vi "Teleop V1.vi"(10 "Match Info":T1={"Autonomous Elapsed Seconds"=0.0, "TeleOp Elapsed Seconds"=567.647, "Disabled Elapsed Seconds"=48.494, "Visited Autonomous"=FALSE, "Visited TeleOp"=TRUE, "Visited Disabled"=TRUE, "Autonomous Settings"={"Autonomous Style"=enum."Independent", "VI Refnum"=refnum}}) -> ()   [LabVIEW 2018]
doc: "This VI is called for each TeleOp packet received from the DS where the robot is not disabled. It is often used to read from the joysticks and update I/O or to update setpoints for timed control loops. It should complete and return within 20 milliseconds or it may miss DS packets."
uses:
  <vilib>/Rock Robotics/WPI/DriverStation/WPI_DriverStationMatch Info.ctl
  <vilib>/Rock Robotics/WPI/Solenoid/WPI_SolenoidValue.ctl
  <vilib>/Rock Robotics/WPI/ThirdParty/Phoenix-LabVIEW/Motor Controller/Controls/CTRE_Phoenix_MotorControl_ControlMode.ctl
  Refnums.vi
  <vilib>/Rock Robotics/Network Tables/NT Write Numeric Array.vi
  <vilib>/Rock Robotics/Network Tables/NT Write Boolean Array.vi
  <vilib>/Rock Robotics/WPI/Solenoid/WPI_SolenoidSetEnum.vi
  <vilib>/Rock Robotics/WPI/ThirdParty/Phoenix-LabVIEW/Motor Controller/Get/CTRE_Phoenix_MotorController_GetQuadratureData.vi
  Various Globals.vi
panel:
  out "Climber Position":dbl=-130.0
  in  "Elevator cargo":dbl=10500.0
  in  "Elevator First Level":dbl=5500.0
  in  "Pivot Under Flat":dbl=1300.0
  in  "Climber Clear 2":dbl=-300.0
  out "Boolean":bool=TRUE
  out "Pivot Position":dbl=64.0
  out "Elevator Position":dbl=439.0
  in  "Random Climber":dbl=2000.0
  in  "Climber Climb":dbl=5500.0
  in  "Elevator Tucked":dbl=500.0
  in  "Pivot Up":dbl
  in  "Elevator Intake":dbl=500.0
  in  "Climber Clear":dbl=1500.0
  in  "Elevator Clearance":dbl=4750.0
  in  "Pivot Intake":dbl=1650.0
  in  "Second level":dbl=14500.0
  in  "First Ball":dbl=7500.0
  in  "Climber Intake":dbl=2700.0
  in  "Climber Up":dbl
  # "Climber Intake \nChanged From\n2800"
  # "<---- Changed From 1700"
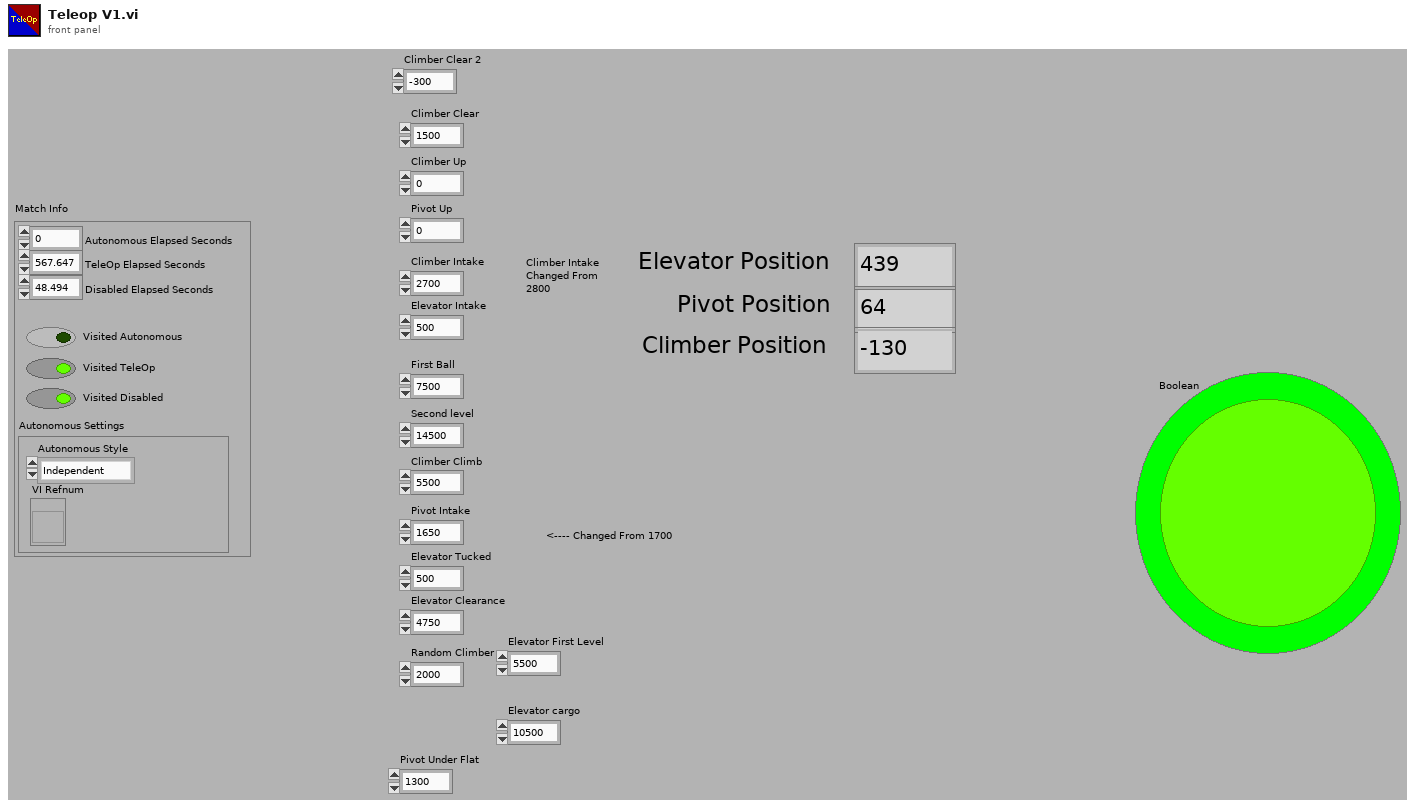
[diagram p1: front panel]
types:
  T1 = typedef "WPI_DriverStationMatch Info.ctl" = cluster{"Autonomous Elapsed Seconds":dbl, "TeleOp Elapsed Seconds":dbl, "Disabled Elapsed Seconds":dbl, "Visited Autonomous":bool, "Visited TeleOp":bool, "Visited Disabled":bool, "Autonomous Settings":cluster{"Autonomous Style":enum16{"Iterative", "Independent"}, "VI Refnum":refnum<vi>}}
  T2 = typedef "WPI_JoystickDevRef.ctl" = cluster{"Device":T3}
  T3 = typedef "WPI_JoystickDeviceEnum.ctl" = enum16{"USB 0", "USB 1", "USB 2", "USB 3", "USB 4", "USB 5"}
  T4 = typedef "WPI_RobotDriveDevRef.ctl" = cluster{"DevStatus":errorcluster, "Motors[]":T5[], "Square Inputs":bool, "Max Output":dbl}
  T5 = typedef "WPI_MotorControlDeviceRef.ctl" = cluster{"DeviceStatus":errorcluster, "Type":T6, "PWM":cluster{"PWM Channel":T7, "DeadBand":T8}, "CAN":cluster{"Device Number":u8, "SetOutput VI Ref":variant, "GetOutput VI Ref":variant, "Enable VI Ref":variant, "Disable VI Ref":variant, "Data":variant}, "Invert":bool, "DIO PWM":cluster{"PWM \"Enable\" Channel":T7, "DIOChannel":T9, "PWM Rate":dbl}}
  T6 = typedef "WPI_MotorControlType.ctl" = enum16{"PWM", "CAN", "DIO PWM"}
  T7 = typedef "FPGA_DIOPWMChannel.ctl" = enum8{"PWM 0", "PWM 1", "PWM 2", "PWM 3", "PWM 4", "PWM 5", "PWM 6", "PWM 7", "PWM 8", "PWM 9", "PWM MXP 0", "PWM MXP 1", "PWM MXP 2", "PWM MXP 3", "PWM MXP 4", "PWM MXP 5", "PWM MXP 6", "PWM MXP 7", "PWM MXP 8", "PWM MXP 9", "Invalid"}
  T8 = typedef "WPI_PWMDeadband.ctl" = cluster{"Name":string, "maxPositivePwm":i32, "minPositivePwm":i32, "centerPwm":i32, "maxNegativePwm":i32, "minNegativePwm":i32, "angularRange":u16}
  T9 = typedef "FPGA_DIOChannel.ctl" = enum8{"DIO 0", "DIO 1", "DIO 2", "DIO 3", "DIO 4", "DIO 5", "DIO 6", "DIO 7", "DIO 8", "DIO 9", "DIO MXP 0", "DIO MXP 1", "DIO MXP 2", "DIO MXP 3", "DIO MXP 4", "DIO MXP 5", "DIO MXP 6", "DIO MXP 7", "DIO MXP 8", "DIO MXP 9", "DIO MXP 10", "DIO MXP 11", "DIO MXP 12", "DIO MXP 13", "DIO MXP 14", "DIO MXP 15", "SPI Port CS1", "SPI Port CS2", "SPI Port CS3", "SPI Port MISO", "SPI Port MOSI", "Invalid"}
  T10 = cluster{"DriveTrain":T4, "LeftDrive":T5, "RightDrive":T5, "Elevator":T5, "Pivot":T5, "Intake":T5, "Right Climber":T5, "Left Climber":T5, "Shooter":T5}
  T11 = typedef "WPI_SolenoidDevRef.ctl" = cluster{"DevStatus":errorcluster, "Pneumatics Control Module":u8, "Forward Solenoid Channel":T12, "Reverse Solenoid Channel":T12}
  T12 = typedef "WPI_SolenoidChannel.ctl" = enum8{"Solenoid 0", "Solenoid 1", "Solenoid 2", "Solenoid 3", "Solenoid 4", "Solenoid 5", "Solenoid 6", "Solenoid 7", "Invalid"}
  T13 = typedef "WPI_CompressorDevRef.ctl" = cluster{"DevStatus":errorcluster, "Pneumatics Control Module":u8}
  T14 = cluster{"DriveShifter":T11, "Ouput":T11, "Compressor":T13, "Climb Piston":T11}
  T15 = typedef "WPI_SolenoidValue.ctl" = enum16{"Off", "On", "Forward", "Reverse"}
  T16 = typedef "WPI_DigitalInputDevRef.ctl" = cluster{"DevStatus":errorcluster, "DIO Channel":T9}
  T17 = typedef "CTRE_Phoenix_MotorControl_ControlMode.ctl" = u16
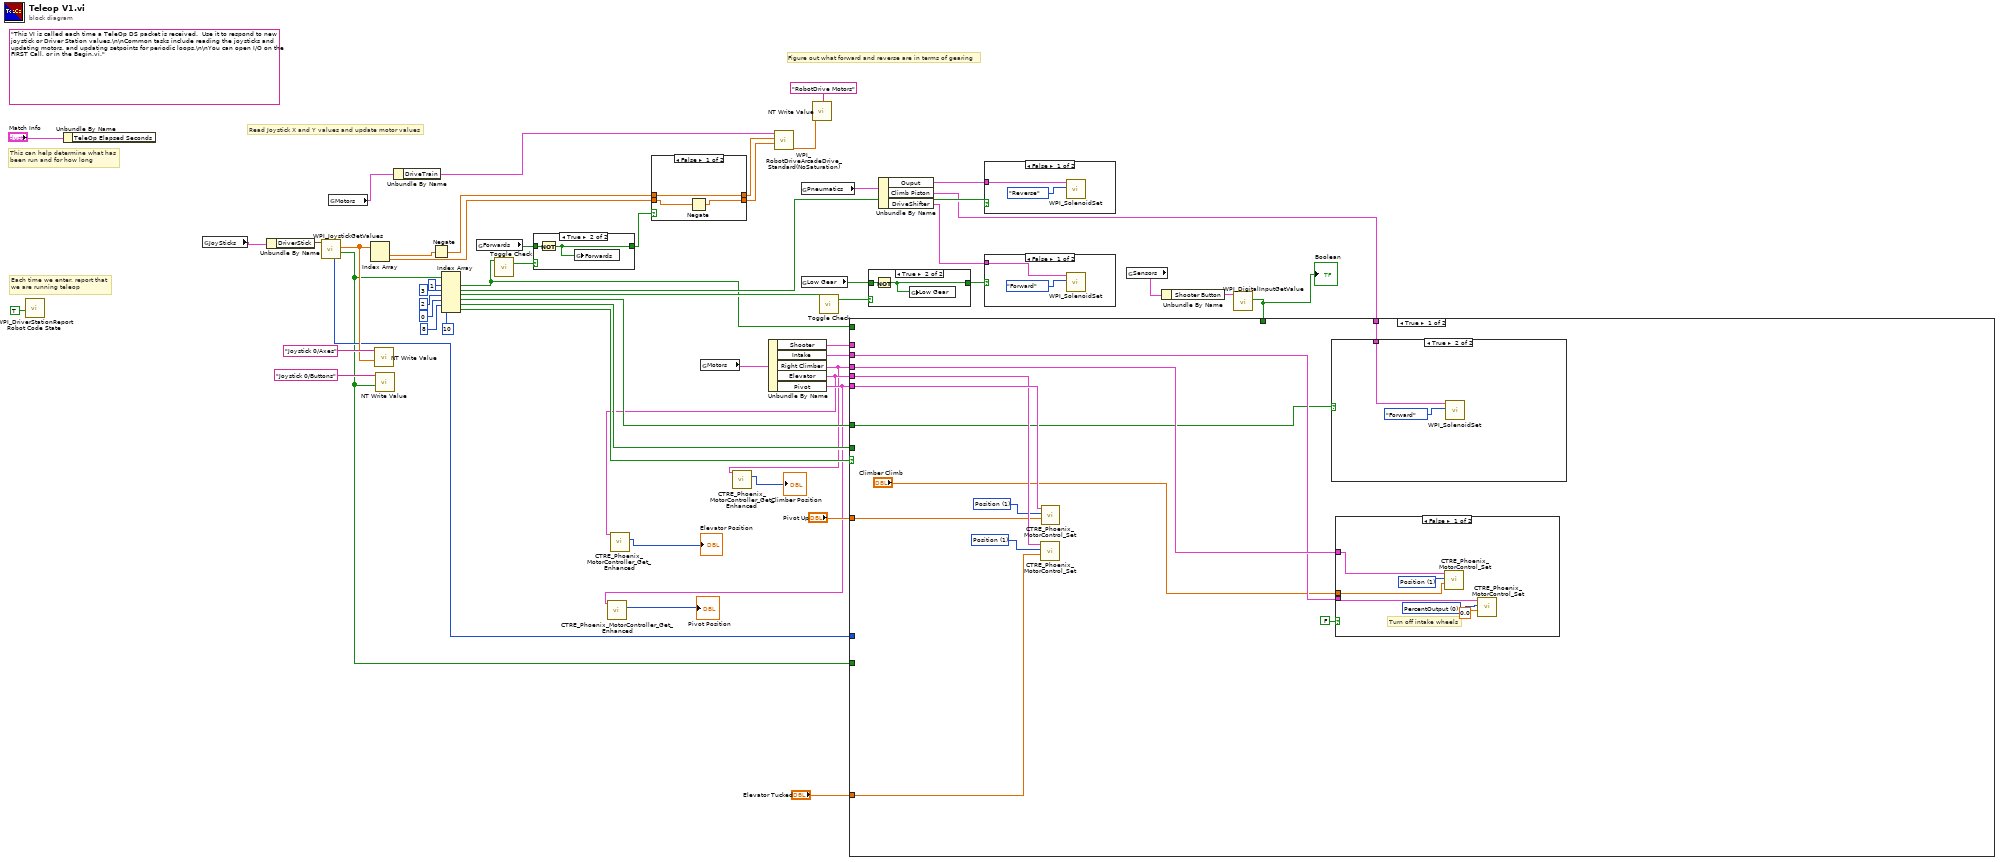
[diagram p0: block diagram]
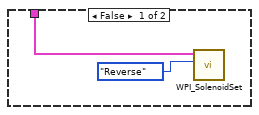
[diagram p2: hidden frame]
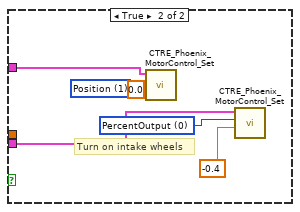
[diagram p3: hidden frame]
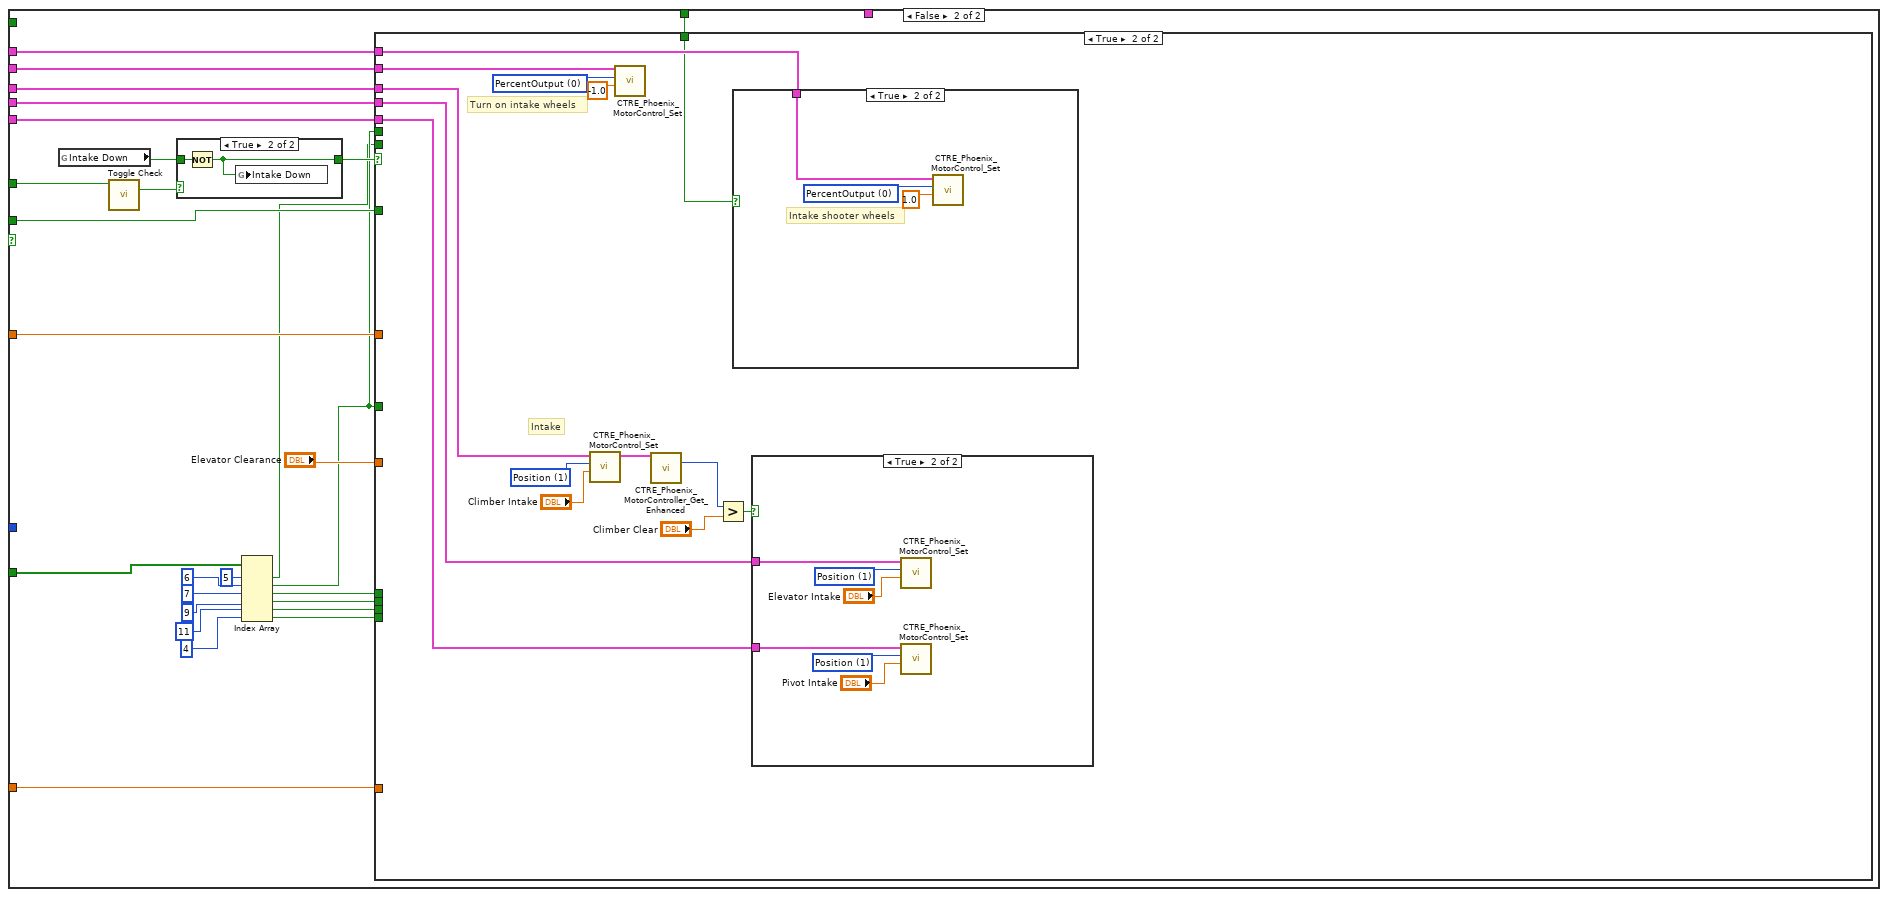
[diagram p4: hidden frame]
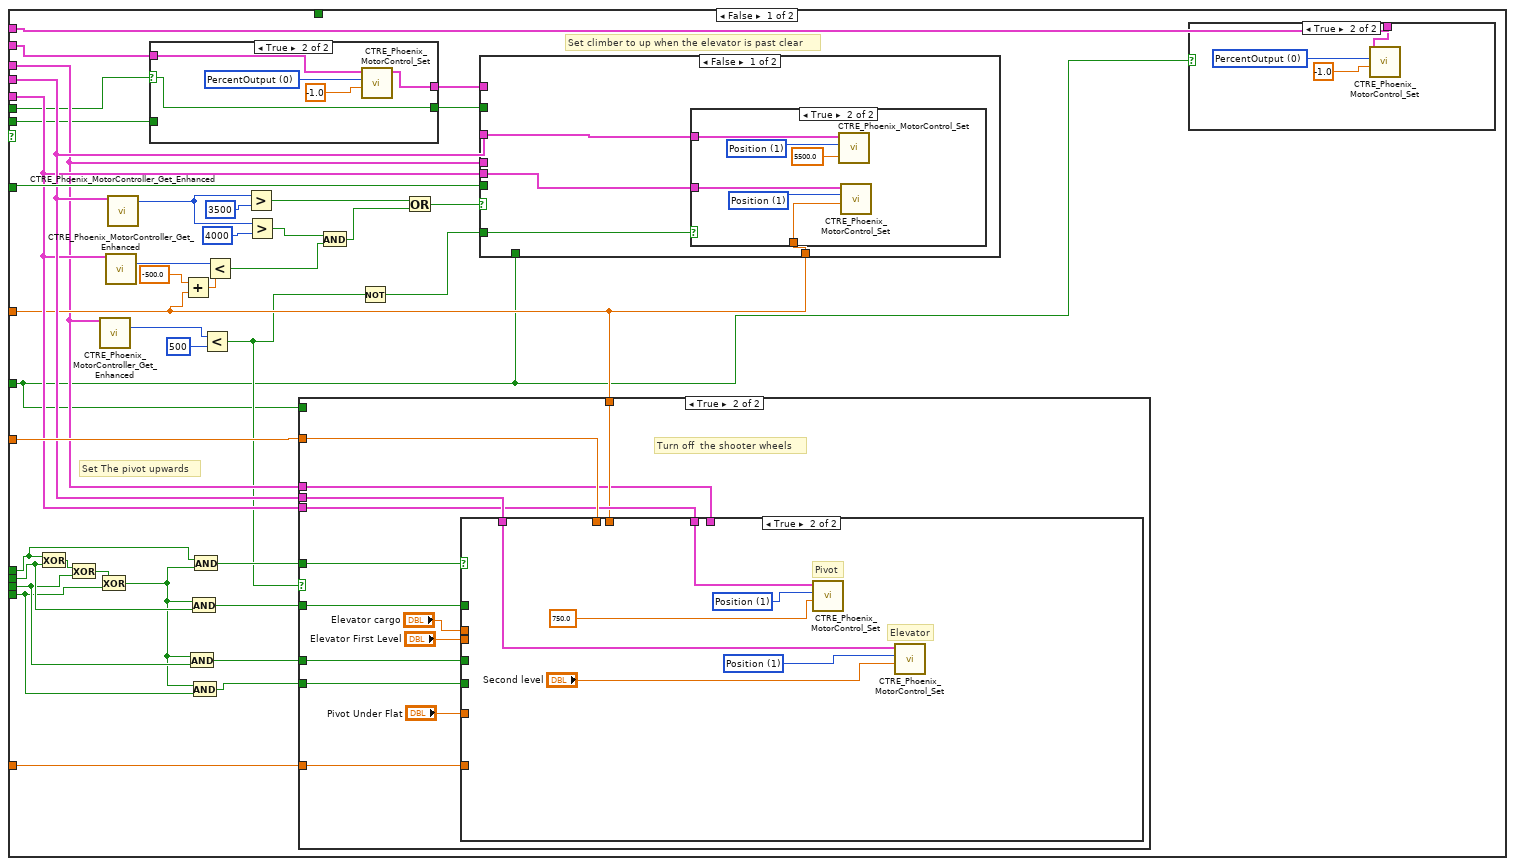
[diagram p6: hidden frame]
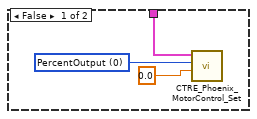
[diagram p7: hidden frame]
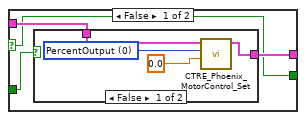
[diagram p8: hidden frame]
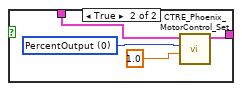
[diagram p9: hidden frame]
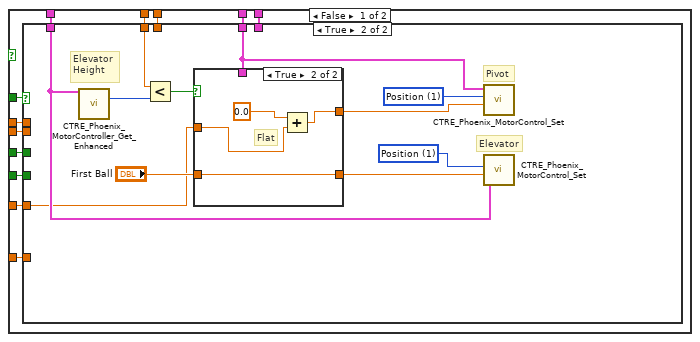
[diagram p11: hidden frame]
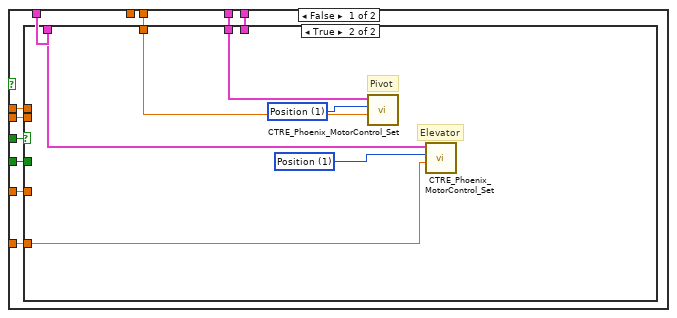
[diagram p12: hidden frame]
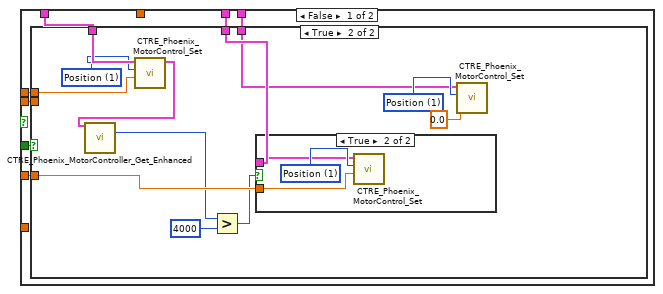
[diagram p13: hidden frame]
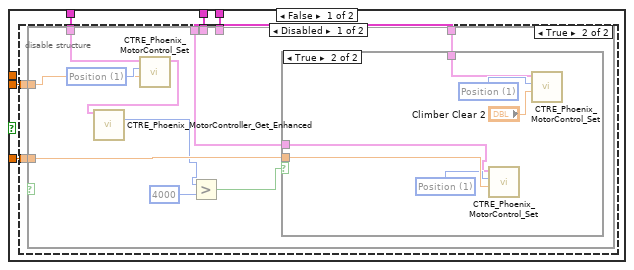
[diagram p14: hidden frame]
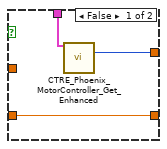
[diagram p19: hidden frame]
diagram:
  (unwired) "This VI is called each time a TeleOp DS packet is received.  Use it to respond to new joystick or Driver Station values.\n\nCommon tasks include reading the joysticks and updating motors, and updating setpoints for periodic loops.\n\nYou can open I/O on the FIRST Call, or in the Begin.vi."
  # "Figure out what forward and reverse are in terms of gearing"
  # "Each time we enter, report that\nwe are running teleop"
  # "This can help determine what has\nbeen run and for how long"
  # "Read Joystick X and Y values and update motor values"
  n1 = call <vilib>:"WPI_DriverStationReport Robot Code State.vi"("TeleOp"=TRUE ("Autonomous")) -> ()  [unwired: 10 in, 1 out]
  n2 = Unbundle By Name("Match Info") -> ()  [unwired: 1 out]
  n3 = global read "Refnums.vi" "JoySticks"() -> (w49:cluster{"DriverStick":T2, "OperatorStick":T2})
  n4 = Unbundle By Name(w49) -> ("DriverStick"=w48:T2)
  n5 = call <vilib>:"WPI_JoystickGetValues.vi"("JoystickDevRef"=w48) -> ("Buttons"=w2:bool[], "Axes"=w50:dbl[], "POVs"=w9:i16[])  [unwired: 6 in, 2 out]
  n6 = global read "Refnums.vi" "Motors"() -> (w45:T10)
  n7 = Index Array(array=w50) -> (element #1=w41:dbl, element #2=w19:dbl)  [unwired: 2 in]
  n8 = call-poly <vilib>:"NT Write Value.vi"("Numeric Array"=w50, "Name"="Joystick 0/Axes") -> ()  [unwired: 9 in, 1 out]
  n9 = call-poly <vilib>:"NT Write Value.vi"("Boolean Array"=w2, "Name"="Joystick 0/Buttons") -> ()  [unwired: 9 in, 1 out]
  n10 = Unbundle By Name(w45) -> ("DriveTrain"=w46:T4)
  n11 = Negate(x=w41) -> (-x=w20:dbl)
  n12 = Index Array(array=w2, index #1=1 ("index"), index #2=3, index #3=2, index #4=0, index #5=8 ("index"), index #6=10 ("index")) -> (element #1=w8:bool, element #2=w33:bool, element #3=w24:bool, element #4=w42:bool, element #5=w28:bool, element #6=w29:bool)
  n13 = global read "Various Globals.vi" "Forwards"() -> (w21:bool)
  n14 = call "Toggle Check.vi"("button in"=w8) -> ("toggled?"=w22:bool)  [unwired: 10 in]
  n15 = case shown="True" w22 {
    tunnel: [w55 w57] -> w1
    tunnel: w21 -> [w55 w56]
    frame False {
    }
    frame True {
      n16 = Not(x=w56) -> (.not. x?=w57:bool)
      n17 = global write "Various Globals.vi" "Forwards"(w57) -> ()
    }
  }
  n18 = case shown="False" w1 {
    tunnel: w20 -> [w60 w62]
    tunnel: w19 -> [w59 w61]
    tunnel: [w60 w62] -> w3
    tunnel: [w58 w61] -> w4
    frame False {
      n19 = Negate(x=w59) -> (-x=w58:dbl)
    }
    frame True {
    }
  }
  n20 = global read "Refnums.vi" "Motors"() -> (w40:T10)
  n21 = Unbundle By Name(w40) -> ("Shooter"=w35:T5, "Intake"=w39:T5, "Right Climber"=w10:T5, "Elevator"=w12:T5, "Pivot"=w17:T5)
  n22 = call-poly <vilib>:"CTRE_Phoenix_MotorController_Get_Enhanced.vi"("PhoenixMotorControlDevRef"=w17) -> ("Quadrature Position"=→"Pivot Position":i32)  [unwired: 11 in, 3 out]
  n23 = call-poly <vilib>:"CTRE_Phoenix_MotorController_Get_Enhanced.vi"("PhoenixMotorControlDevRef"=w12) -> ("Quadrature Position"=→"Elevator Position":i32)  [unwired: 11 in, 3 out]
  n24 = call-poly <vilib>:"CTRE_Phoenix_MotorController_Get_Enhanced.vi"("PhoenixMotorControlDevRef"=w10) -> ("Quadrature Position"=→"Climber Position":i32)  [unwired: 11 in, 3 out]
  n25 = call <vilib>:"WPI_RobotDriveArcadeDrive_Standard(NoSaturation).vi"("Y axis value"=w4, "X axis value"=w3, "RobotDriveDevRef"=w46) -> ("Motor Values"=w44:dbl[])  [unwired: 1 in, 7 out]
  n26 = global read "Refnums.vi" "Pneumatics"() -> (w47:T14)
  n27 = global read "Various Globals.vi" "Low Gear"() -> (w26:bool)
  n28 = call-poly <vilib>:"NT Write Value.vi"("Numeric Array"=w44, "Name"="RobotDrive Motors") -> ()  [unwired: 9 in, 1 out]
  n29 = call "Toggle Check.vi"("button in"=w24) -> ("toggled?"=w27:bool)  [unwired: 10 in]
  n30 = case shown="True" w27 {
    tunnel: [w63 w65] -> w25
    tunnel: w26 -> [w63 w64]
    frame False {
    }
    frame True {
      n31 = Not(x=w64) -> (.not. x?=w65:bool)
      n32 = global write "Various Globals.vi" "Low Gear"(w65) -> ()
    }
  }
  n33 = Unbundle By Name(w47) -> ("Ouput"=w34:T11, "Climb Piston"=w6:T11, "DriveShifter"=w7:T11)
  n34 = case shown="False" w33 {
    tunnel: w34 -> [w66 w68]
    frame False {
      n35 = call-poly <vilib>:"WPI_SolenoidSet.vi"("Value"=WPI_SolenoidValue."Reverse", "SolenoidDevRef"=w66) -> ()  [unwired: 8 in, 2 out]
    }
    frame True {
      n36 = call-poly <vilib>:"WPI_SolenoidSet.vi"("Value"=WPI_SolenoidValue."Forward", "SolenoidDevRef"=w68) -> ()  [unwired: 8 in, 2 out]
    }
  }
  n37 = case shown="False" w25 {
    tunnel: w7 -> [w70 w72]
    frame False {
      n38 = call-poly <vilib>:"WPI_SolenoidSet.vi"("Value"=WPI_SolenoidValue."Forward", "SolenoidDevRef"=w70) -> ()  [unwired: 8 in, 2 out]
    }
    frame True {
      n39 = call-poly <vilib>:"WPI_SolenoidSet.vi"("Value"=WPI_SolenoidValue."Reverse", "SolenoidDevRef"=w72) -> ()  [unwired: 8 in, 2 out]
    }
  }
  n40 = global read "Refnums.vi" "Sensors"() -> (w14:cluster{"Shooter Button":T16})
  n41 = Unbundle By Name(w14) -> ("Shooter Button"=w13:T16)
  n42 = call <vilib>:"WPI_DigitalInputGetValue.vi"("DigitalInputDevRef"=w13) -> ("Value"=w15:bool)  [unwired: 8 in, 2 out]
  "Boolean" <- w15
  n43 = case shown="True" w29 {
    tunnel: w42 -> [w75 w128]
    tunnel: w39 -> [w82 w106]
    tunnel: w10 -> [w84 w109]
    tunnel: w12 -> [w83 w125]
    tunnel: w2 -> [_ w123]
    tunnel: w17 -> [w85 w116]
    tunnel: w35 -> [_ w115]
    tunnel: w15 -> [_ w113]
    tunnel: "Pivot Up" -> [w80 w112]
    tunnel: w28 -> [_ w110]
    tunnel: w9 -> [_ _]
    tunnel: w8 -> [_ _]
    tunnel: w6 -> [w76 _]
    tunnel: "Elevator Tucked" -> [w79 w104]
    frame True {
      w77 = T17 1 items=["PercentOutput"=0, "Position"=1, "Velocity"=2, "Current"=3, "Follower"=5, "MotionProfile"=6, "MotionMagic"=7, "MotionProfileArc"=10, "Disabled"=15] ("Control Mode")
      w78 = T17 1 items=["PercentOutput"=0, "Position"=1, "Velocity"=2, "Current"=3, "Follower"=5, "MotionProfile"=6, "MotionMagic"=7, "MotionProfileArc"=10, "Disabled"=15] ("Control Mode")
      n44 = call <vilib>:"CTRE_Phoenix_MotorControl_Set.vi"("Output"=w79, "Control Mode"=w78, "PhoenixMotorControlDevRef"=w83) -> ()  [unwired: 7 in, 2 out]
      n45 = call <vilib>:"CTRE_Phoenix_MotorControl_Set.vi"("Output"=w80, "Control Mode"=w77, "PhoenixMotorControlDevRef"=w85) -> ()  [unwired: 7 in, 2 out]
      n46 = case shown="True" w75 {
        tunnel: w76 -> [w86 w88]
        frame False {
          n47 = call-poly <vilib>:"WPI_SolenoidSet.vi"("Value"=WPI_SolenoidValue."Reverse", "SolenoidDevRef"=w86) -> ()  [unwired: 8 in, 2 out]
        }
        frame True {
          n48 = call-poly <vilib>:"WPI_SolenoidSet.vi"("Value"=WPI_SolenoidValue."Forward", "SolenoidDevRef"=w88) -> ()  [unwired: 8 in, 2 out]
        }
      }
      n49 = case shown="False" FALSE {
        tunnel: w82 -> [w93 w99]
        tunnel: w84 -> [w91 w97]
        tunnel: "Climber Climb" -> [w90 _]
        frame False {
          w92 = T17 1 items=["PercentOutput"=0, "Position"=1, "Velocity"=2, "Current"=3, "Follower"=5, "MotionProfile"=6, "MotionMagic"=7, "MotionProfileArc"=10, "Disabled"=15] ("Control Mode")
          w94 = T17 0 items=["PercentOutput"=0, "Position"=1, "Velocity"=2, "Current"=3, "Follower"=5, "MotionProfile"=6, "MotionMagic"=7, "MotionProfileArc"=10, "Disabled"=15] ("Control Mode")
          # "Turn off intake wheels"
          n50 = call <vilib>:"CTRE_Phoenix_MotorControl_Set.vi"("Output"=w90, "Control Mode"=w92, "PhoenixMotorControlDevRef"=w91) -> ()  [unwired: 7 in, 2 out]
          n51 = call <vilib>:"CTRE_Phoenix_MotorControl_Set.vi"("Output"=0.0, "Control Mode"=w94, "PhoenixMotorControlDevRef"=w93) -> ()  [unwired: 7 in, 2 out]
        }
        frame True {
          w98 = T17 1 items=["PercentOutput"=0, "Position"=1, "Velocity"=2, "Current"=3, "Follower"=5, "MotionProfile"=6, "MotionMagic"=7, "MotionProfileArc"=10, "Disabled"=15] ("Control Mode")
          w100 = T17 0 items=["PercentOutput"=0, "Position"=1, "Velocity"=2, "Current"=3, "Follower"=5, "MotionProfile"=6, "MotionMagic"=7, "MotionProfileArc"=10, "Disabled"=15] ("Control Mode")
          # "Turn on intake wheels"
          n52 = call <vilib>:"CTRE_Phoenix_MotorControl_Set.vi"("Output"=0.0, "Control Mode"=w98, "PhoenixMotorControlDevRef"=w97) -> ()  [unwired: 7 in, 2 out]
          n53 = call <vilib>:"CTRE_Phoenix_MotorControl_Set.vi"("Output"=-0.4, "Control Mode"=w100, "PhoenixMotorControlDevRef"=w99) -> ()  [unwired: 7 in, 2 out]
        }
      }
    }
    frame False {
      n54 = global read "Various Globals.vi" "Intake Down"() -> (w126:bool)
      n55 = call "Toggle Check.vi"("button in"=w128) -> ("toggled?"=w127:bool)  [unwired: 10 in]
      n56 = case shown="True" w127 {
        tunnel: [w129 w131] -> w124
        tunnel: w126 -> [w129 w130]
        frame False {
        }
        frame True {
          n57 = Not(x=w130) -> (.not. x?=w131:bool)
          n58 = global write "Various Globals.vi" "Intake Down"(w131) -> ()
        }
      }
      n59 = Index Array(array=w123, index #1=5 ("index"), index #2=6 ("index"), index #3=7 ("index"), index #4=9 ("index"), index #5=11 ("index"), index #6=4 ("index")) -> (element #1=w102:bool, element #2=w105:bool, element #3=w119:bool, element #4=w118:bool, element #5=w117:bool, element #6=w107:bool)
      n60 = case shown="True" w124 {
        tunnel: w109 -> [w144 w341]
        tunnel: w106 -> [w138 w339]
        tunnel: w115 -> [w139 w338]
        tunnel: w125 -> [w162 w331]
        tunnel: w116 -> [w160 w330]
        tunnel: w119 -> [w149 _]
        tunnel: w118 -> [w148 _]
        tunnel: w117 -> [w147 _]
        tunnel: w105 -> [w140 _]
        tunnel: w113 -> [_ w329]
        tunnel: "Elevator Clearance" -> [w168 _]
        tunnel: w112 -> [w157 _]
        tunnel: w110 -> [w167 _]
        tunnel: w107 -> [w146 _]
        tunnel: w105 -> [w137 _]
        tunnel: w104 -> [w136 _]
        tunnel: w102 -> [w133 _]
        frame False {
          # "Set The pivot upwards"
          # "Set climber to up when the elevator is past clear"
          n61 = Exclusive Or(1:w148, 2:w149) -> (0:w151:bool)
          n62 = Exclusive Or(1:w147, 2:w151) -> (0:w150:bool)
          n63 = Exclusive Or(1:w146, 2:w150) -> (0:w134:bool)
          n64 = call-poly <vilib>:"CTRE_Phoenix_MotorController_Get_Enhanced.vi"("PhoenixMotorControlDevRef"=w144) -> ("Quadrature Position"=w171:i32)  [unwired: 11 in, 3 out]
          n65 = call-poly <vilib>:"CTRE_Phoenix_MotorController_Get_Enhanced.vi"("PhoenixMotorControlDevRef"=w160) -> ("Quadrature Position"=w159:i32)  [unwired: 11 in, 3 out]
          n66 = call-poly <vilib>:"CTRE_Phoenix_MotorController_Get_Enhanced.vi"("PhoenixMotorControlDevRef"=w162) -> ("Quadrature Position"=w161:i32)  [unwired: 11 in, 3 out]
          n67 = case shown="True" w137 {
            selector: w137 -> [w178 w190]
            tunnel: w138 -> [w181 w192]
            tunnel: [w180 w191] -> w135
            tunnel: w133 -> [w179 _]
            tunnel: [w178 w190] -> w132
            frame False {
              n68 = case shown="False" w179 {
                tunnel: w181 -> [w183 w188]
                tunnel: [w182 w186] -> w180
                frame False {
                  w184 = T17 0 items=["PercentOutput"=0, "Position"=1, "Velocity"=2, "Current"=3, "Follower"=5, "MotionProfile"=6, "MotionMagic"=7, "MotionProfileArc"=10, "Disabled"=15] ("Control Mode")
                  n69 = call <vilib>:"CTRE_Phoenix_MotorControl_Set.vi"("Output"=0.0, "Control Mode"=w184, "PhoenixMotorControlDevRef"=w183) -> ("PhoenixMotorControlDevRef"=w182:T5)  [unwired: 7 in, 1 out]
                }
                frame True {
                  w187 = T17 0 items=["PercentOutput"=0, "Position"=1, "Velocity"=2, "Current"=3, "Follower"=5, "MotionProfile"=6, "MotionMagic"=7, "MotionProfileArc"=10, "Disabled"=15] ("Control Mode")
                  n70 = call <vilib>:"CTRE_Phoenix_MotorControl_Set.vi"("Output"=1.0, "Control Mode"=w187, "PhoenixMotorControlDevRef"=w188) -> ("PhoenixMotorControlDevRef"=w186:T5)  [unwired: 7 in, 1 out]
                }
              }
            }
            frame True {
              w193 = T17 0 items=["PercentOutput"=0, "Position"=1, "Velocity"=2, "Current"=3, "Follower"=5, "MotionProfile"=6, "MotionMagic"=7, "MotionProfileArc"=10, "Disabled"=15] ("Control Mode")
              n71 = call <vilib>:"CTRE_Phoenix_MotorControl_Set.vi"("Output"=-1.0, "Control Mode"=w193, "PhoenixMotorControlDevRef"=w192) -> ("PhoenixMotorControlDevRef"=w191:T5)  [unwired: 7 in, 1 out]
            }
          }
          n72 = Add(x=-500.0, y=w157) -> (x+y=w156:dbl)
          n73 = And(x=w134, y=w147) -> (x .and. y?=w154:bool)
          n74 = And(x=w134, y=w148) -> (x .and. y?=w153:bool)
          n75 = And(x=w134, y=w146) -> (x .and. y?=w145:bool)
          n76 = And(x=w149, y=w134) -> (x .and. y?=w152:bool)
          n77 = Less?(x=w171, y=500) -> (x < y?=w141:bool)
          n78 = Less?(x=w159, y=w156) -> (x < y?=w158:bool)
          n79 = Greater?(x=w161, y=3500) -> (0:w165:bool)
          n80 = Greater?(x=w161, y=4000) -> (0:w163:bool)
          n81 = case shown="True" w141 {
            tunnel: w140 -> [_ _]
            tunnel: w168 -> [_ w207]
            tunnel: w162 -> [_ w206]
            tunnel: w160 -> [_ w205]
            tunnel: w157 -> [_ w204]
            tunnel: w154 -> [_ w203]
            tunnel: w153 -> [_ w202]
            tunnel: w152 -> [_ w201]
            tunnel: w145 -> [_ w200]
            tunnel: w144 -> [_ w199]
            tunnel: w136 -> [_ w195]
            frame False {
            }
            frame True {
              # "Turn off  the shooter wheels"
              n82 = case shown="True" w201 {
                tunnel: w202 -> [w219 _]
                tunnel: w203 -> [w218 _]
                tunnel: w206 -> [w217 w303]
                tunnel: w207 -> [w216 _]
                tunnel: w205 -> [w215 w302]
                tunnel: w204 -> [w214 _]
                tunnel: w200 -> [w213 _]
                tunnel: w199 -> [w212 _]
                tunnel: "Elevator First Level" -> [w211 _]
                tunnel: "Pivot Under Flat" -> [w210 _]
                tunnel: "Elevator cargo" -> [w209 _]
                tunnel: w195 -> [w208 _]
                frame False {
                  n83 = case shown="True" w219 {
                    tunnel: w218 -> [w229 _]
                    tunnel: w217 -> [w228 w289]
                    tunnel: w216 -> [_ w292]
                    tunnel: w215 -> [w227 w288]
                    tunnel: w214 -> [w226 _]
                    tunnel: w213 -> [w225 _]
                    tunnel: w212 -> [w224 _]
                    tunnel: w211 -> [w223 _]
                    tunnel: w210 -> [w222 w284]
                    tunnel: w209 -> [w221 _]
                    tunnel: w208 -> [w220 _]
                    frame False {
                      n84 = case shown="True" w229 {
                        tunnel: w228 -> [w234 w280]
                        tunnel: w227 -> [w232 w281]
                        tunnel: w226 -> [_ w279]
                        tunnel: w225 -> [w236 _]
                        tunnel: w224 -> [w235 _]
                        tunnel: w223 -> [w233 _]
                        tunnel: w222 -> [w231 _]
                        tunnel: w221 -> [w230 _]
                        tunnel: w220 -> [_ w278]
                        frame False {
                          n85 = case shown="True" w236 {
                            tunnel: w235 -> [w239 w268]
                            tunnel: w234 -> [w241 w274]
                            tunnel: w233 -> [w240 _]
                            tunnel: w232 -> [w237 w271]
                            tunnel: w231 -> [w238 w270]
                            tunnel: w230 -> [_ w273]
                            frame False {
                              n86 = disable-structure shown="Disabled" {
                                disable-tunnel: w241 -> [w246 _]
                                disable-tunnel: w240 -> [w245 _]
                                disable-tunnel: w239 -> [w244 _]
                                disable-tunnel: w238 -> [w243 _]
                                disable-tunnel: w237 -> [w242 _]
                                frame Disabled {
                                n87 = case shown="True" {
                                selector: _ -> [_ _]
                                tunnel: w244 -> [_ _]
                                tunnel: w246 -> [_ w255]
                                tunnel: w245 -> [_ w254]
                                tunnel: w242 -> [_ _]
                                tunnel: w244 -> [_ w253]
                                tunnel: w243 -> [_ w252]
                                tunnel: w242 -> [_ w251]
                                frame False {
                                }
                                frame True {
                                w256 = T17 1 items=["PercentOutput"=0, "Position"=1, "Velocity"=2, "Current"=3, "Follower"=5, "MotionProfile"=6, "MotionMagic"=7, "MotionProfileArc"=10, "Disabled"=15] ("Control Mode")
                                n88 = call <vilib>:"CTRE_Phoenix_MotorControl_Set.vi"("Output"=w254, "Control Mode"=w256, "PhoenixMotorControlDevRef"=w255) -> ("PhoenixMotorControlDevRef"=w250:T5)  [unwired: 7 in, 1 out]
                                n89 = call-poly <vilib>:"CTRE_Phoenix_MotorController_Get_Enhanced.vi"("PhoenixMotorControlDevRef"=w250) -> ("Quadrature Position"=w249:i32)  [unwired: 11 in, 3 out]
                                n90 = Greater?(x=w249, y=4000) -> (0:w247:bool)
                                n91 = case shown="True" w247 {
                                tunnel: w253 -> [_ w260]
                                tunnel: w252 -> [_ w259]
                                tunnel: w251 -> [_ w257]
                                frame False {
                                }
                                frame True {
                                w258 = T17 1 items=["PercentOutput"=0, "Position"=1, "Velocity"=2, "Current"=3, "Follower"=5, "MotionProfile"=6, "MotionMagic"=7, "MotionProfileArc"=10, "Disabled"=15] ("Control Mode")
                                w261 = T17 1 items=["PercentOutput"=0, "Position"=1, "Velocity"=2, "Current"=3, "Follower"=5, "MotionProfile"=6, "MotionMagic"=7, "MotionProfileArc"=10, "Disabled"=15] ("Control Mode")
                                n92 = call <vilib>:"CTRE_Phoenix_MotorControl_Set.vi"("Output"=w259, "Control Mode"=w258, "PhoenixMotorControlDevRef"=w257) -> ()  [unwired: 7 in, 2 out]
                                n93 = call <vilib>:"CTRE_Phoenix_MotorControl_Set.vi"("Output"="Climber Clear 2", "Control Mode"=w261, "PhoenixMotorControlDevRef"=w260) -> ()  [unwired: 7 in, 2 out]
                                }
                                }
                                }
                                }
                                }
                                frame Enabled {
                                }
                              }
                            }
                            frame True {
                              w269 = T17 1 items=["PercentOutput"=0, "Position"=1, "Velocity"=2, "Current"=3, "Follower"=5, "MotionProfile"=6, "MotionMagic"=7, "MotionProfileArc"=10, "Disabled"=15] ("Control Mode")
                              w272 = T17 1 items=["PercentOutput"=0, "Position"=1, "Velocity"=2, "Current"=3, "Follower"=5, "MotionProfile"=6, "MotionMagic"=7, "MotionProfileArc"=10, "Disabled"=15] ("Control Mode")
                              n94 = call <vilib>:"CTRE_Phoenix_MotorControl_Set.vi"("Output"=w273, "Control Mode"=w272, "PhoenixMotorControlDevRef"=w274) -> ("PhoenixMotorControlDevRef"=w265:T5)  [unwired: 7 in, 1 out]
                              n95 = call-poly <vilib>:"CTRE_Phoenix_MotorController_Get_Enhanced.vi"("PhoenixMotorControlDevRef"=w265) -> ("Quadrature Position"=w264:i32)  [unwired: 11 in, 3 out]
                              n96 = Greater?(x=w264, y=4000) -> (0:w263:bool)
                              n97 = case shown="True" w263 {
                                tunnel: w271 -> [_ w276]
                                tunnel: w270 -> [_ w275]
                                frame False {
                                }
                                frame True {
                                w277 = T17 1 items=["PercentOutput"=0, "Position"=1, "Velocity"=2, "Current"=3, "Follower"=5, "MotionProfile"=6, "MotionMagic"=7, "MotionProfileArc"=10, "Disabled"=15] ("Control Mode")
                                n98 = call <vilib>:"CTRE_Phoenix_MotorControl_Set.vi"("Output"=w275, "Control Mode"=w277, "PhoenixMotorControlDevRef"=w276) -> ()  [unwired: 7 in, 2 out]
                                }
                              }
                              n99 = call <vilib>:"CTRE_Phoenix_MotorControl_Set.vi"("Output"=0.0, "Control Mode"=w269, "PhoenixMotorControlDevRef"=w268) -> ()  [unwired: 7 in, 2 out]
                            }
                          }
                        }
                        frame True {
                          w283 = T17 1 items=["PercentOutput"=0, "Position"=1, "Velocity"=2, "Current"=3, "Follower"=5, "MotionProfile"=6, "MotionMagic"=7, "MotionProfileArc"=10, "Disabled"=15] ("Control Mode")
                          w282 = T17 1 items=["PercentOutput"=0, "Position"=1, "Velocity"=2, "Current"=3, "Follower"=5, "MotionProfile"=6, "MotionMagic"=7, "MotionProfileArc"=10, "Disabled"=15] ("Control Mode")
                          # "Elevator"
                          # "Pivot"
                          n100 = call <vilib>:"CTRE_Phoenix_MotorControl_Set.vi"("Output"=w279, "Control Mode"=w282, "PhoenixMotorControlDevRef"=w281) -> ()  [unwired: 7 in, 2 out]
                          n101 = call <vilib>:"CTRE_Phoenix_MotorControl_Set.vi"("Output"=w278, "Control Mode"=w283, "PhoenixMotorControlDevRef"=w280) -> ()  [unwired: 7 in, 2 out]
                        }
                      }
                    }
                    frame True {
                      w291 = T17 1 items=["PercentOutput"=0, "Position"=1, "Velocity"=2, "Current"=3, "Follower"=5, "MotionProfile"=6, "MotionMagic"=7, "MotionProfileArc"=10, "Disabled"=15] ("Control Mode")
                      w290 = T17 1 items=["PercentOutput"=0, "Position"=1, "Velocity"=2, "Current"=3, "Follower"=5, "MotionProfile"=6, "MotionMagic"=7, "MotionProfileArc"=10, "Disabled"=15] ("Control Mode")
                      # "Elevator"
                      # "Pivot"
                      # "Elevator \nHeight"
                      n102 = call-poly <vilib>:"CTRE_Phoenix_MotorController_Get_Enhanced.vi"("PhoenixMotorControlDevRef"=w289) -> ("Quadrature Position"=w293:i32)  [unwired: 11 in, 3 out]
                      n103 = Less?(x=w292, y=w293) -> (x < y?=w285:bool)
                      n104 = case shown="True" w285 {
                        tunnel: [w296 w298] -> w287
                        tunnel: "First Ball" -> [w297 w301]
                        tunnel: [w297 w301] -> w286
                        tunnel: w288 -> [w295 _]
                        tunnel: w284 -> [_ w299]
                        frame False {
                          n105 = call-poly <vilib>:"CTRE_Phoenix_MotorController_Get_Enhanced.vi"("PhoenixMotorControlDevRef"=w295) -> ("Quadrature Position"=w296:i32)  [unwired: 11 in, 3 out]
                        }
                        frame True {
                          # "Flat"
                          n106 = Add(x=0.0, y=w299) -> (x+y=w298:dbl)
                        }
                      }
                      n107 = call <vilib>:"CTRE_Phoenix_MotorControl_Set.vi"("Output"=w287, "Control Mode"=w290, "PhoenixMotorControlDevRef"=w288) -> ()  [unwired: 7 in, 2 out]
                      n108 = call <vilib>:"CTRE_Phoenix_MotorControl_Set.vi"("Output"=w286, "Control Mode"=w291, "PhoenixMotorControlDevRef"=w289) -> ()  [unwired: 7 in, 2 out]
                    }
                  }
                }
                frame True {
                  w306 = T17 1 items=["PercentOutput"=0, "Position"=1, "Velocity"=2, "Current"=3, "Follower"=5, "MotionProfile"=6, "MotionMagic"=7, "MotionProfileArc"=10, "Disabled"=15] ("Control Mode")
                  w304 = T17 1 items=["PercentOutput"=0, "Position"=1, "Velocity"=2, "Current"=3, "Follower"=5, "MotionProfile"=6, "MotionMagic"=7, "MotionProfileArc"=10, "Disabled"=15] ("Control Mode")
                  # "Elevator"
                  # "Pivot"
                  n109 = call <vilib>:"CTRE_Phoenix_MotorControl_Set.vi"("Output"=750.0 ("Pivot Up"), "Control Mode"=w304, "PhoenixMotorControlDevRef"=w302) -> ()  [unwired: 7 in, 2 out]
                  n110 = call <vilib>:"CTRE_Phoenix_MotorControl_Set.vi"("Output"="Second level", "Control Mode"=w306, "PhoenixMotorControlDevRef"=w303) -> ()  [unwired: 7 in, 2 out]
                }
              }
            }
          }
          n111 = And(x=w163, y=w158) -> (x .and. y?=w142:bool)
          n112 = Not(x=w141) -> (.not. x?=w143:bool)
          n113 = Or(x=w165, y=w142) -> (x .or. y?=w166:bool)
          n114 = case shown="False" w166 {
            tunnel: w162 -> [w311 _]
            tunnel: w157 -> [w310 _]
            tunnel: w144 -> [_ w322]
            tunnel: w160 -> [w309 _]
            tunnel: w143 -> [w308 _]
            tunnel: w167 -> [_ w320]
            tunnel: w140 -> [_ w321]
            tunnel: w135 -> [_ w319]
            tunnel: w132 -> [_ w318]
            frame False {
              n115 = case shown="True" w308 {
                tunnel: w311 -> [_ w317]
                tunnel: w310 -> [_ w313]
                tunnel: w309 -> [_ w312]
                frame False {
                }
                frame True {
                  w314 = T17 1 items=["PercentOutput"=0, "Position"=1, "Velocity"=2, "Current"=3, "Follower"=5, "MotionProfile"=6, "MotionMagic"=7, "MotionProfileArc"=10, "Disabled"=15] ("Control Mode")
                  w316 = T17 1 items=["PercentOutput"=0, "Position"=1, "Velocity"=2, "Current"=3, "Follower"=5, "MotionProfile"=6, "MotionMagic"=7, "MotionProfileArc"=10, "Disabled"=15] ("Control Mode")
                  n116 = call <vilib>:"CTRE_Phoenix_MotorControl_Set.vi"("Output"=5500.0, "Control Mode"=w316, "PhoenixMotorControlDevRef"=w317) -> ()  [unwired: 7 in, 2 out]
                  n117 = call <vilib>:"CTRE_Phoenix_MotorControl_Set.vi"("Output"=w313, "Control Mode"=w314, "PhoenixMotorControlDevRef"=w312) -> ()  [unwired: 7 in, 2 out]
                }
              }
            }
            frame True {
              n118 = case shown="False" w320 {
                tunnel: w322 -> [w325 w326]
                tunnel: w321 -> [_ _]
                tunnel: w319 -> [_ _]
                tunnel: w318 -> [_ _]
                frame True {
                  w324 = T17 1 items=["PercentOutput"=0, "Position"=1, "Velocity"=2, "Current"=3, "Follower"=5, "MotionProfile"=6, "MotionMagic"=7, "MotionProfileArc"=10, "Disabled"=15] ("Control Mode")
                  n119 = call <vilib>:"CTRE_Phoenix_MotorControl_Set.vi"("Output"="Random Climber", "Control Mode"=w324, "PhoenixMotorControlDevRef"=w325) -> ()  [unwired: 7 in, 2 out]
                }
                frame False {
                  w328 = T17 1 items=["PercentOutput"=0, "Position"=1, "Velocity"=2, "Current"=3, "Follower"=5, "MotionProfile"=6, "MotionMagic"=7, "MotionProfileArc"=10, "Disabled"=15] ("Control Mode")
                  n120 = call <vilib>:"CTRE_Phoenix_MotorControl_Set.vi"("Output"="Climber Up", "Control Mode"=w328, "PhoenixMotorControlDevRef"=w326) -> ()  [unwired: 7 in, 2 out]
                }
              }
            }
          }
          n121 = case shown="True" w140 {
            tunnel: w139 -> [w174 w175]
            frame False {
              w172 = T17 0 items=["PercentOutput"=0, "Position"=1, "Velocity"=2, "Current"=3, "Follower"=5, "MotionProfile"=6, "MotionMagic"=7, "MotionProfileArc"=10, "Disabled"=15] ("Control Mode")
              n122 = call <vilib>:"CTRE_Phoenix_MotorControl_Set.vi"("Output"=0.0, "Control Mode"=w172, "PhoenixMotorControlDevRef"=w174) -> ()  [unwired: 7 in, 2 out]
            }
            frame True {
              w176 = T17 0 items=["PercentOutput"=0, "Position"=1, "Velocity"=2, "Current"=3, "Follower"=5, "MotionProfile"=6, "MotionMagic"=7, "MotionProfileArc"=10, "Disabled"=15] ("Control Mode")
              n123 = call <vilib>:"CTRE_Phoenix_MotorControl_Set.vi"("Output"=-1.0, "Control Mode"=w176, "PhoenixMotorControlDevRef"=w175) -> ()  [unwired: 7 in, 2 out]
            }
          }
        }
        frame True {
          w340 = T17 0 items=["PercentOutput"=0, "Position"=1, "Velocity"=2, "Current"=3, "Follower"=5, "MotionProfile"=6, "MotionMagic"=7, "MotionProfileArc"=10, "Disabled"=15] ("Control Mode")
          w342 = T17 1 items=["PercentOutput"=0, "Position"=1, "Velocity"=2, "Current"=3, "Follower"=5, "MotionProfile"=6, "MotionMagic"=7, "MotionProfileArc"=10, "Disabled"=15] ("Control Mode")
          # "Intake"
          # "Turn on intake wheels"
          n124 = call <vilib>:"CTRE_Phoenix_MotorControl_Set.vi"("Output"="Climber Intake", "Control Mode"=w342, "PhoenixMotorControlDevRef"=w341) -> ("PhoenixMotorControlDevRef"=w335:T5)  [unwired: 7 in, 1 out]
          n125 = call <vilib>:"CTRE_Phoenix_MotorControl_Set.vi"("Output"=-1.0, "Control Mode"=w340, "PhoenixMotorControlDevRef"=w339) -> ()  [unwired: 7 in, 2 out]
          n126 = call-poly <vilib>:"CTRE_Phoenix_MotorController_Get_Enhanced.vi"("PhoenixMotorControlDevRef"=w335) -> ("Quadrature Position"=w334:i32)  [unwired: 11 in, 3 out]
          n127 = Greater?(x=w334, y="Climber Clear") -> (0:w332:bool)
          n128 = case shown="True" w329 {
            selector: w329 -> [w343 _]
            tunnel: w338 -> [w344 w348]
            frame False {
              w346 = T17 0 items=["PercentOutput"=0, "Position"=1, "Velocity"=2, "Current"=3, "Follower"=5, "MotionProfile"=6, "MotionMagic"=7, "MotionProfileArc"=10, "Disabled"=15] ("Control Mode")
              # "Intake shooter wheels"
              n129 = global write "Various Globals.vi" "Intake Down"(w343) -> ()
              n130 = call <vilib>:"CTRE_Phoenix_MotorControl_Set.vi"("Output"=0.0, "Control Mode"=w346, "PhoenixMotorControlDevRef"=w344) -> ()  [unwired: 7 in, 2 out]
            }
            frame True {
              w349 = T17 0 items=["PercentOutput"=0, "Position"=1, "Velocity"=2, "Current"=3, "Follower"=5, "MotionProfile"=6, "MotionMagic"=7, "MotionProfileArc"=10, "Disabled"=15] ("Control Mode")
              # "Intake shooter wheels"
              n131 = call <vilib>:"CTRE_Phoenix_MotorControl_Set.vi"("Output"=1.0, "Control Mode"=w349, "PhoenixMotorControlDevRef"=w348) -> ()  [unwired: 7 in, 2 out]
            }
          }
          n132 = case shown="True" w332 {
            tunnel: w331 -> [_ w355]
            tunnel: w330 -> [_ w354]
            frame False {
            }
            frame True {
              w352 = T17 1 items=["PercentOutput"=0, "Position"=1, "Velocity"=2, "Current"=3, "Follower"=5, "MotionProfile"=6, "MotionMagic"=7, "MotionProfileArc"=10, "Disabled"=15] ("Control Mode")
              w353 = T17 1 items=["PercentOutput"=0, "Position"=1, "Velocity"=2, "Current"=3, "Follower"=5, "MotionProfile"=6, "MotionMagic"=7, "MotionProfileArc"=10, "Disabled"=15] ("Control Mode")
              n133 = call <vilib>:"CTRE_Phoenix_MotorControl_Set.vi"("Output"="Elevator Intake", "Control Mode"=w353, "PhoenixMotorControlDevRef"=w355) -> ()  [unwired: 7 in, 2 out]
              n134 = call <vilib>:"CTRE_Phoenix_MotorControl_Set.vi"("Output"="Pivot Intake", "Control Mode"=w352, "PhoenixMotorControlDevRef"=w354) -> ()  [unwired: 7 in, 2 out]
            }
          }
        }
      }
    }
  }
